vi "示例 6.vi"() -> ()   [LabVIEW 2021]
panel:
  out "dt":u32
  in  "Boolean":bool
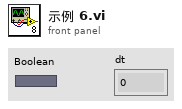
[diagram p1: front panel]
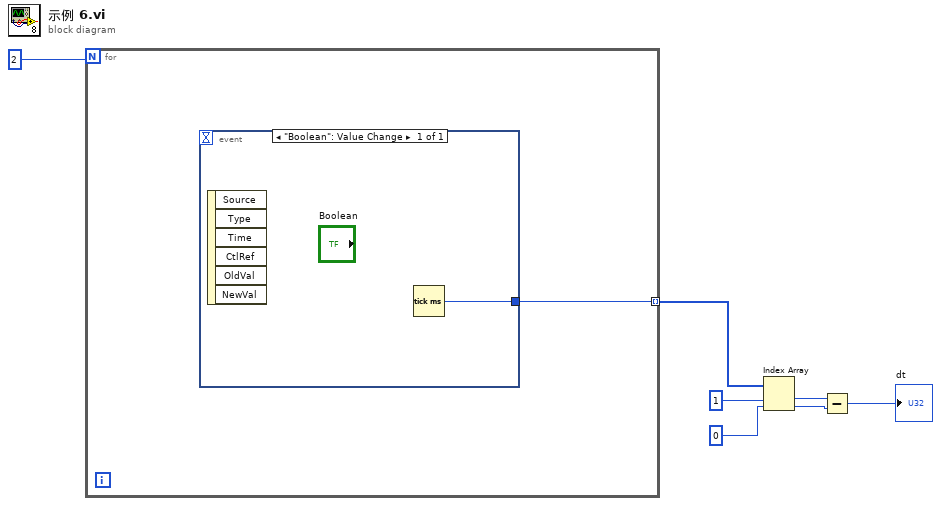
[diagram p0: block diagram]
diagram:
  n1 = for {
    N: 2 -> [_]
    tunnel: [w8] -> w4 mode=indexing
    n2 = event shown="[0] \"Boolean\": Value Change" {
      selector: _ -> [_]
      dyn-events: _ -> [_]
      timeout: _ -> [_]
      tunnel: [w9] -> w8
      event "Boolean": Value Change {
        n3 = event-data() -> ()  [unwired: 1 in, 6 out]
        n4 = Tick Count (ms)() -> (millisecond timer value=w9:u32)
      }
    }
  }
  n5 = Index Array(array=w4, index #1=1, index #2=0) -> (element #1=w3:u32, element #2=w2:u32)
  n6 = Subtract(x=w3, y=w2) -> (x-y=→"dt":u32)
